vi "p5Segudir_Brazo3.vi"() -> ()   [LabVIEW 2017]
uses:
  <vilib>/LabVIEW Interface for Arduino/Type Defs/Board Type.ctl
  <vilib>/LabVIEW Interface for Arduino/LabVIEW Interface for Arduino.lvlib
panel:
  out "x+y 2":dbl
  out "x+y":dbl
  out "s? t:f 2":u8
  in  "Home":bool
  out "s? t:f":u8
  in  "VISA resource":refnum<visa-resource-name>
  in  "Board Type":T1
  out "Servo 0":u8(knob) scale=0.0..180.0
  out "Servo 1":u8(knob) scale=0.0..180.0
  out "new picture 2":picture
  out "error y":dbl
  out "error x":dbl
  out "x":dbl
  out "y":dbl
  in  "Slide 2":dbl(slide) scale=0.0..255.0
  out "new picture":picture
  in  "Stop (F)":bool
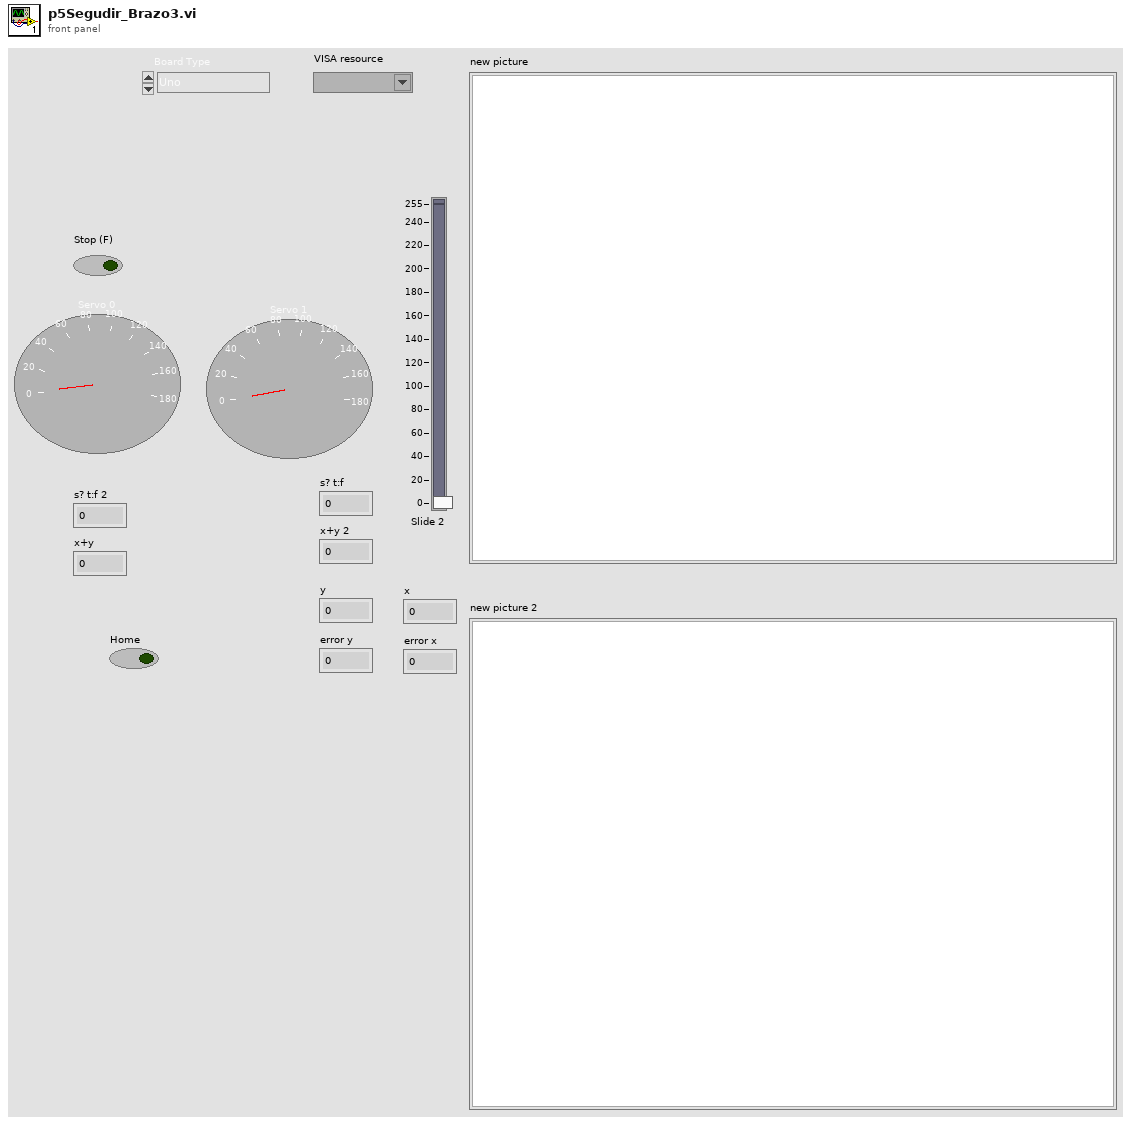
[diagram p1: front panel]
types:
  T1 = typedef "LabVIEW Interface for Arduino.lvlib/Board Type.ctl" = enum16{"Uno", "Dimuelanove w/Atmega 328", "Mega 2560"}
  T2 = typedef "LabVIEW Interface for Arduino.lvlib/Arduino Resource.ctl" = cluster{"VISA resource":refnum<visa-resource-name>, "Board Type":T1, "Connection Type":enum8{"USB / Serial"}, "Bytes Per Packet (15)":u8}
  T3 = typedef "IMAQ Image.ctl" = refnum<image>
  T4 = typedef "imagedata.ctl" = cluster{"image type":i32, "image depth":i32, "image":u8[], "mask":u8[], "colors":u32[], "Rectangle":cluster{"left":i16, "top":i16, "right":i16, "bottom":i16}}
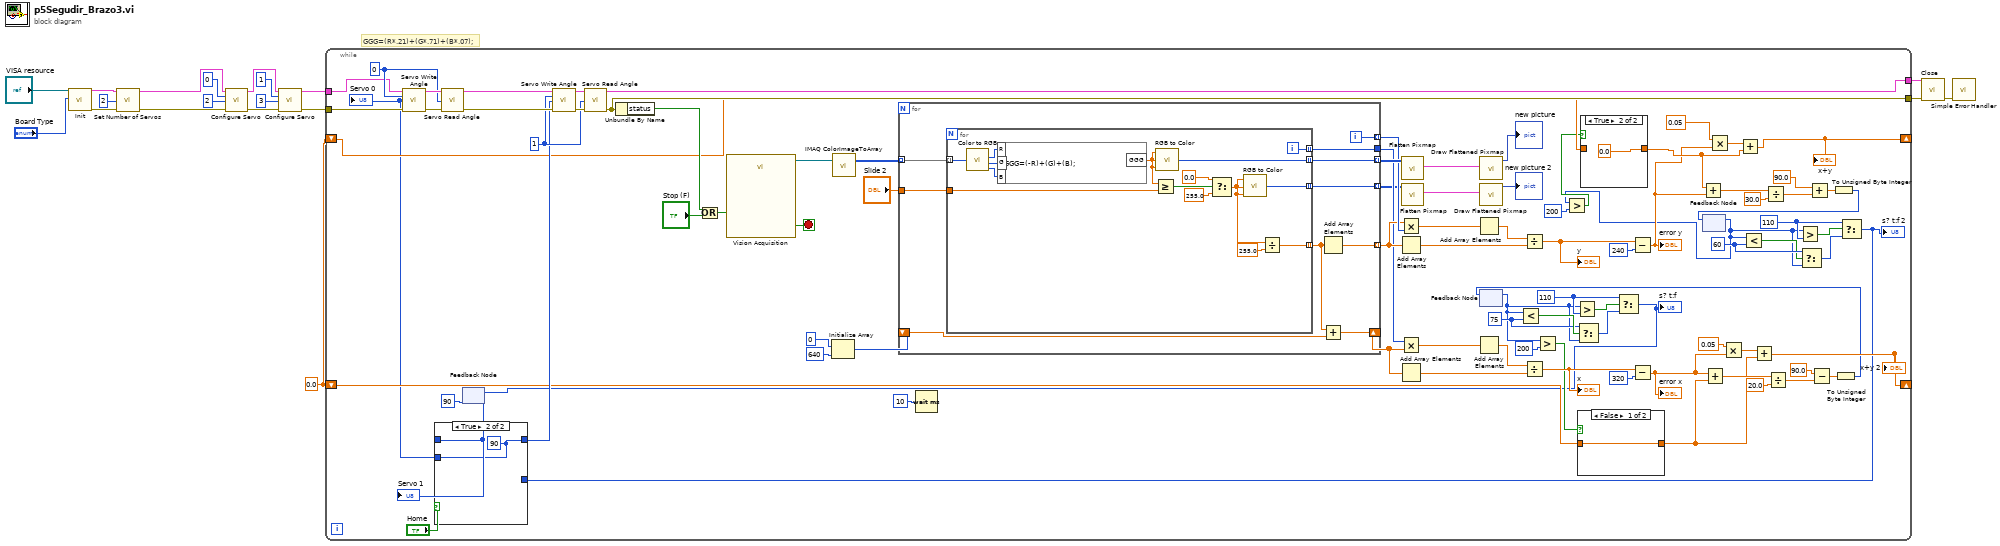
[diagram p0: block diagram]
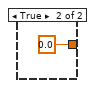
[diagram p3: hidden frame]
diagram:
  w1 = 0.0
  # "GGG=(R*.21)+(G*.71)+(B*.07);"
  n1 = call <vilib>:"Init.vi"("VISA resource"="VISA resource", "Board Type (Uno)"="Board Type") -> ("Arduino Resource"=w8:T2, "error out"=w9:errorcluster)  [unwired: 16 in]
  n2 = call <vilib>:"Set Number of Servos.vi"("Arduino Resource"=w8, "Number Of Servos (1)"=u8 2 ("Number of Servos"), "error in"=w9) -> ("Arduino Resource"=w11:T2, "error out"=w12:errorcluster)  [unwired: 11 in]
  n3 = call <vilib>:"Configure Servo.vi"("Arduino Resource"=w11, "Servo Number (0)"=u8 0 ("Servo Number"), "DIO Pin (2)"=u8 2 ("Servo Number"), "error in"=w12) -> ("Arduino Resource"=w13:T2, "error out"=w14:errorcluster)  [unwired: 10 in]
  n4 = call <vilib>:"Configure Servo.vi"("Arduino Resource"=w13, "Servo Number (0)"=u8 1 ("Servo Number"), "DIO Pin (2)"=u8 3 ("Servo Number"), "error in"=w14) -> ("Arduino Resource"=w5:T2, "error out"=w4:errorcluster)  [unwired: 10 in]
  n5 = while {
    tunnel: w5 -> [w73]
    tunnel: w4 -> [w72]
    tunnel: [w71] -> w3
    tunnel: [w70] -> w2
    shift-right: [w53] -> _
    shift-left: w1 -> [w49]
    shift-right: [w39] -> _
    shift-left: w1 -> [w38]
    stop <- w109 stop-if-true
    w29 = u8 60 ("y")
    w28 = u8 110 ("y")
    w61 = u8 75 ("y")
    w62 = u8 110 ("y")
    w75 = u8 1 ("Servo Number")
    w74 = u8 0 ("Servo Number")
    n6 = feedback #1(u8 90 ("y")) -> (w47:u8)
    "Servo 1" <- w47
    n7 = Initialize Array(0 ("element"), 640 ("dimension size")) -> (w96:i32[])
    n8 = Wait (ms)(milliseconds to wait=u32 10) -> ()  [unwired: 1 out]
    n9 = feedback #2() -> (w43:u8)  [unwired: 1 in]
    n10 = Less?(x=w43, y=w61) -> (x < y?=w65:bool)
    n11 = Greater?(x=w43, y=u8 200) -> (0:w52:bool)
    n12 = Greater?(x=w43, y=w62) -> (0:w66:bool)
    n13 = Select(t=w61, s=w65, f=w43) -> (s? t:f=w60:u8)
    n14 = case shown="False" w52 {
      tunnel: w49 -> [w112 _]
      tunnel: [w112 0.0] -> w48
      frame False {
      }
      frame True {
      }
    }
    n15 = Select(t=w62, s=w66, f=w60) -> (s? t:f=w46:u8)
    "s? t:f" <- w46
    n16 = feedback-in #1(w46) -> ()
    n17 = feedback #3() -> (w24:u8)  [unwired: 1 in]
    n18 = Greater?(x=w24, y=u8 200) -> (0:w36:bool)
    n19 = case shown="True" w36 {
      tunnel: w38 -> [w110 _]
      tunnel: [w110 0.0] -> w32
      frame False {
      }
      frame True {
      }
    }
    n20 = Less?(x=w24, y=w29) -> (x < y?=w27:bool)
    n21 = Greater?(x=w24, y=w28) -> (0:w26:bool)
    n22 = Select(t=w29, s=w27, f=w24) -> (s? t:f=w30:u8)
    n23 = Select(t=w28, s=w26, f=w30) -> (s? t:f=w23:u8)
    "s? t:f 2" <- w23
    n24 = case shown="True" "Home" {
      tunnel: [w115 w116] -> w51
      tunnel: w47 -> [w115 _]
      tunnel: w23 -> [w114 _]
      tunnel: [w114 w116] -> w22
      frame False {
      }
      frame True {
        w116 = u8 90 ("y")
      }
    }
    "Servo 0" <- w22
    n25 = call <vilib>:"Servo Write Angle.vi"("Arduino Resource"=w73, "Servo Number"=w74, "Angle (Degrees)"=w22, "error in"=w72) -> ("Arduino Resource"=w76:T2, "error out"=w77:errorcluster)  [unwired: 10 in]
    n26 = call <vilib>:"Servo Read Angle.vi"("Arduino Resource"=w76, "Servo Number"=w74, "error in"=w77) -> ("Arduino Resource"=w81:T2, "error out"=w78:errorcluster)  [unwired: 10 in, 1 out]
    n27 = call <vilib>:"Servo Write Angle.vi"("Arduino Resource"=w81, "Servo Number"=w75, "Angle (Degrees)"=w51, "error in"=w78) -> ("Arduino Resource"=w80:T2, "error out"=w79:errorcluster)  [unwired: 10 in]
    n28 = call <vilib>:"Servo Read Angle.vi"("Arduino Resource"=w80, "Servo Number"=w75, "error in"=w79) -> ("Arduino Resource"=w71:T2, "error out"=w70:errorcluster)  [unwired: 10 in, 1 out]
    n29 = Unbundle By Name(w70) -> ("status"=w82:bool)
    n30 = Or(x=w82, y="Stop (F)") -> (x .or. y?=w69:bool)
    n31 = call "Vision Acquisition"("Stop (F)"=w69) -> ("Image Out"=w108:T3, "Stopped"=w109:bool)  [unwired: 24 in, 1 out]
    n32 = call "IMAQ ColorImageToArray"("Image"=w108) -> ("Image Pixels (U32)"=w84:u32[][])  [unwired: 3 in, 2 out]
    n33 = for {
      tunnel: w84 -> [w126] mode=indexing
      tunnel: [w125] -> w107 mode=indexing
      tunnel: "Slide 2" -> [w124]
      tunnel: [w123] -> w100 mode=indexing
      tunnel: [w122] -> w103 mode=indexing
      shift-right: [w119] -> w91
      shift-left: w96 -> [w120]
      tunnel: [w118] -> w95
      tunnel: [w117] -> w83 mode=indexing
      i -> [w122]
      n34 = for {
        tunnel: w126 -> [w132] mode=indexing
        tunnel: [w141] -> w125 mode=indexing
        tunnel: w124 -> [w138]
        tunnel: [w136] -> w121 mode=indexing
        tunnel: [w135] -> w118 mode=indexing
        tunnel: [w129] -> w117 mode=indexing
        i -> [w135]
        n35 = call <vilib>:"Color to RGB.vi"("Color"=w132) -> ("R"=w128:u8, "G"=w134:u8, "B"=w133:u8)  [unwired: 1 out]
        n36 = formula code="GGG=(-R)+(G)+(B);"("R"=w128, "G"=w134, "B"=w133) -> ("GGG"=w127:dbl)
        n37 = Greater Or Equal?(x=w127, y=w138) -> (x >= y?=w131:bool)
        n38 = call <vilib>:"RGB to Color.vi"("B"=w127, "G"=w127, "R"=w127) -> ("Color"=w141:u32)
        n39 = Select(t=0.0, s=w131, f=255.0) -> (s? t:f=w130:dbl)
        n40 = call <vilib>:"RGB to Color.vi"("B"=w130, "G"=w130, "R"=w130) -> ("Color"=w129:u32)
        n41 = Divide(x=w130, y=255.0) -> (x/y=w136:dbl)
      }
      n42 = Add Array Elements(numeric array=w121) -> (sum=w123:dbl)
      n43 = Add(x=w121, y=w120) -> (x+y=w119:dbl[])
    }
    n44 = Multiply(x=w100, y=w103) -> (x*y=w102:dbl[])
    n45 = Add Array Elements(numeric array=w100) -> (sum=w99:dbl)
    n46 = Multiply(x=w95, y=w91) -> (x*y=w92:dbl[])
    n47 = Add Array Elements(numeric array=w91) -> (sum=w94:dbl)
    n48 = call <vilib>:"Flatten Pixmap.vi"("24-bit pixmap"=w107) -> ("image data"=w106:T4)  [unwired: 10 in]
    n49 = call <vilib>:"Flatten Pixmap.vi"("24-bit pixmap"=w83) -> ("image data"=w85:T4)  [unwired: 10 in]
    n50 = Add Array Elements(numeric array=w102) -> (sum=w101:dbl)
    n51 = Add Array Elements(numeric array=w92) -> (sum=w93:dbl)
    n52 = call <vilib>:"Draw Flattened Pixmap.vi"("image data"=w106) -> ("new picture"=→"new picture":picture)  [unwired: 8 in]
    n53 = call <vilib>:"Draw Flattened Pixmap.vi"("image data"=w85) -> ("new picture"=→"new picture 2":picture)  [unwired: 8 in]
    n54 = Divide(x=w101, y=w99) -> (x/y=w89:dbl)
    "y" <- w89
    n55 = Divide(x=w93, y=w94) -> (x/y=w87:dbl)
    "x" <- w87
    n56 = Subtract(x=w89, y=240) -> (x-y=w31:dbl)
    "error y" <- w31
    n57 = Subtract(x=w87, y=320) -> (x-y=w55:dbl)
    "error x" <- w55
    n58 = Add(x=w32, y=w31) -> (x+y=w34:dbl)
    n59 = Add(x=w55, y=w48) -> (x+y=w56:dbl)
    n60 = Multiply(x=0.05, y=w31) -> (x*y=w41:dbl)
    n61 = Multiply(x=0.05, y=w55) -> (x*y=w54:dbl)
    n62 = Add(x=w41, y=w32) -> (x+y=w39:dbl)
    "x+y" <- w39
    n63 = Add(x=w54, y=w48) -> (x+y=w53:dbl)
    "x+y 2" <- w53
    n64 = Divide(x=w34, y=30.0) -> (x/y=w20:dbl)
    n65 = Divide(x=w56, y=20.0) -> (x/y=w67:dbl)
    n66 = Add(x=90.0, y=w20) -> (x+y=w35:dbl)
    n67 = Subtract(x=90.0, y=w67) -> (x-y=w45:dbl)
    n68 = To Unsigned Byte Integer(number=w35) -> (unsigned 8bit integer=w25:u8)
    n69 = feedback-in #3(w25) -> ()
    n70 = To Unsigned Byte Integer(number=w45) -> (unsigned 8bit integer=w44:u8)
    n71 = feedback-in #2(w44) -> ()
  }
  n72 = call <vilib>:"Close.vi"("Arduino Resource"=w3, "error in"=w2) -> ("error out"=w19:errorcluster)  [unwired: 13 in]
  n73 = call <vilib>:"Simple Error Handler.vi"("error in (no error)"=w19) -> ()  [unwired: 4 in, 5 out]
